vi "Impedance_Single_Meas.vi"(11 "Test Params Cluster":T1={"Test Freq. (Hz)"=1702.3933752476319, "Output Signal Amplitude\nVolts Pk"=0.1, "Sampling Time (s)"=0.01, "Sampling Rate (Hz)"=250000.0, "Output Channel"="Dev3/ao0", "Current Channel"="Dev3/ai1", "Voltage Channel"="Dev3/ai0", "Trigger Channel"="/Dev3/ao/StartTrigger", "Number of runs"=5}) -> (0 "Current Complex":cdb=0.1092230559688666-0.017870132117080606i, 1 "Voltage Complex":cdb=-0.17452167799153867-1.07754869267134i, 2 "Time domain Current":waveform(dbl)(graph)={"t0"=timestamp(3724535126.9386544 s since 1904-01-01), "dt"=3.999999999999989e-06, "Y"=array[2500 elements], "attributes"=variant("NI_ChannelName"=variant(string "Dev3/ai1"), "NI_UnitDescription"=variant(string "Volts"))}, 3 "Time domain Voltage":waveform(dbl)(graph)={"t0"=timestamp(3724535127.000671 s since 1904-01-01), "dt"=3.999999999999989e-06, "Y"=array[2500 elements], "attributes"=variant("NI_ChannelName"=variant(string "Dev3/ai0"), "NI_UnitDescription"=variant(string "Volts"))})   [LabVIEW 2020]
uses:
  <vilib>/measure/NI_MABase.lvlib
  <vilib>/DAQmx/configure/timing.llb/DAQmx Timing (Sample Clock).vi
  <vilib>/DAQmx/create/channels.llb/DAQmx Create Channel (AI-Voltage-Basic).vi
  <vilib>/DAQmx/read.llb/DAQmx Read (Analog 1D Wfm NChan NSamp).vi
  <vilib>/DAQmx/configure/trigger.llb/DAQmx Start Trigger (Digital Edge).vi
  <vilib>/DAQmx/create/channels.llb/DAQmx Create Channel (AO-Voltage-Basic).vi
  <vilib>/DAQmx/write.llb/DAQmx Write (Analog Wfm 1Chan NSamp).vi
  <vilib>/measure/NI_MAPro.lvlib
  <vilib>/measure/matone.llb/Extract Single Tone Information 1 Chan.vi
panel:
  out "Test Freq. (Hz)":dbl=1702.3933752476319
  out "Mag Current":dbl=0.1106752798824565
  in  "Use LabView\nSignal Detect":bool=TRUE
  out "detected phase (Rad)":dbl=4.551821517545998
  out "detected amplitude":dbl=1.0915901250774929 format="%.2p"
  in  "search (+/- % of Fsampl.)":dbl
  in  "advanced search":T2={"approx freq. (optional)"=-1.0, "search (+/- % of Fsampl.)"=5.0} {"search (+/- % of Fsampl.)" format="%0.2p"; "approx freq. (optional)" format="%0.2p"}
  out "Detected Time domain Current 2":waveform(dbl)(graph)={"t0"=timestamp(2.12 s since 1904-01-01), "dt"=4e-06, "Y"=array[2500 elements]}
  out "Detected Time domain Voltage 2":waveform(dbl)(graph)={"t0"=timestamp(2.13 s since 1904-01-01), "dt"=4e-06, "Y"=array[2500 elements]}
  out "detected frequency 2":dbl=1700.0000000000045 format="%.2p"
  out "detected frequency":dbl=1700.0000000000045 format="%.2p"
  out "Current phase (deg)":dbl=-0.16217447631966198 format="%.2p"
  out "Voltage phase (deg)":dbl=260.8001620522193 format="%.2p"
  in  "CurentRangeMax":dbl=5.0 format="%0.2f"
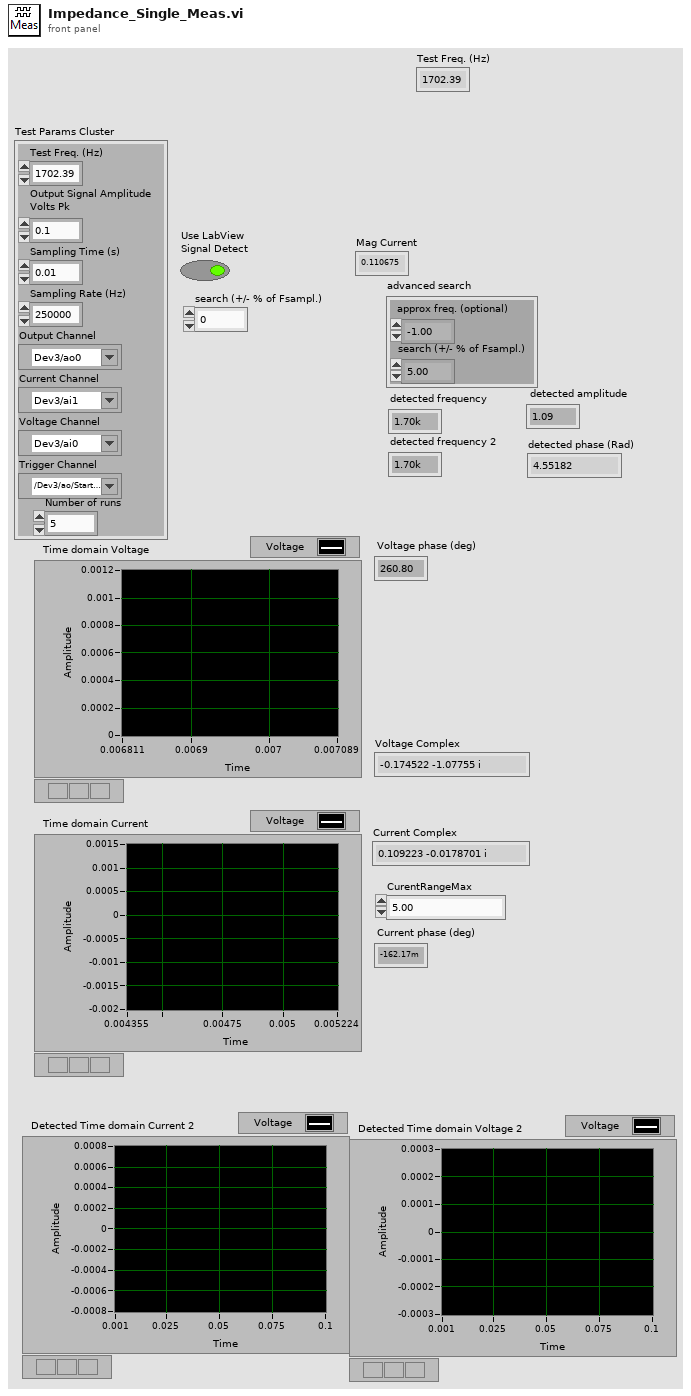
[diagram p1: front panel]
types:
  T1 = cluster{"Test Freq. (Hz)":dbl, "Output Signal Amplitude\nVolts Pk":dbl, "Sampling Time (s)":dbl, "Sampling Rate (Hz)":dbl, "Output Channel":tag, "Current Channel":tag, "Voltage Channel":tag, "Trigger Channel":tag, "Number of runs":i32}
  T2 = cluster{"approx freq. (optional)":dbl, "search (+/- % of Fsampl.)":dbl}
  T3 = enum32{"none", "input signal", "detected signal", "residual signal"}
  T4 = cluster{"exported time signal":waveform(dbl), "exported spectrum (dB)":cluster{"f0":dbl, "df":dbl, "dB Spectrum (Hann)":dbl[]}}
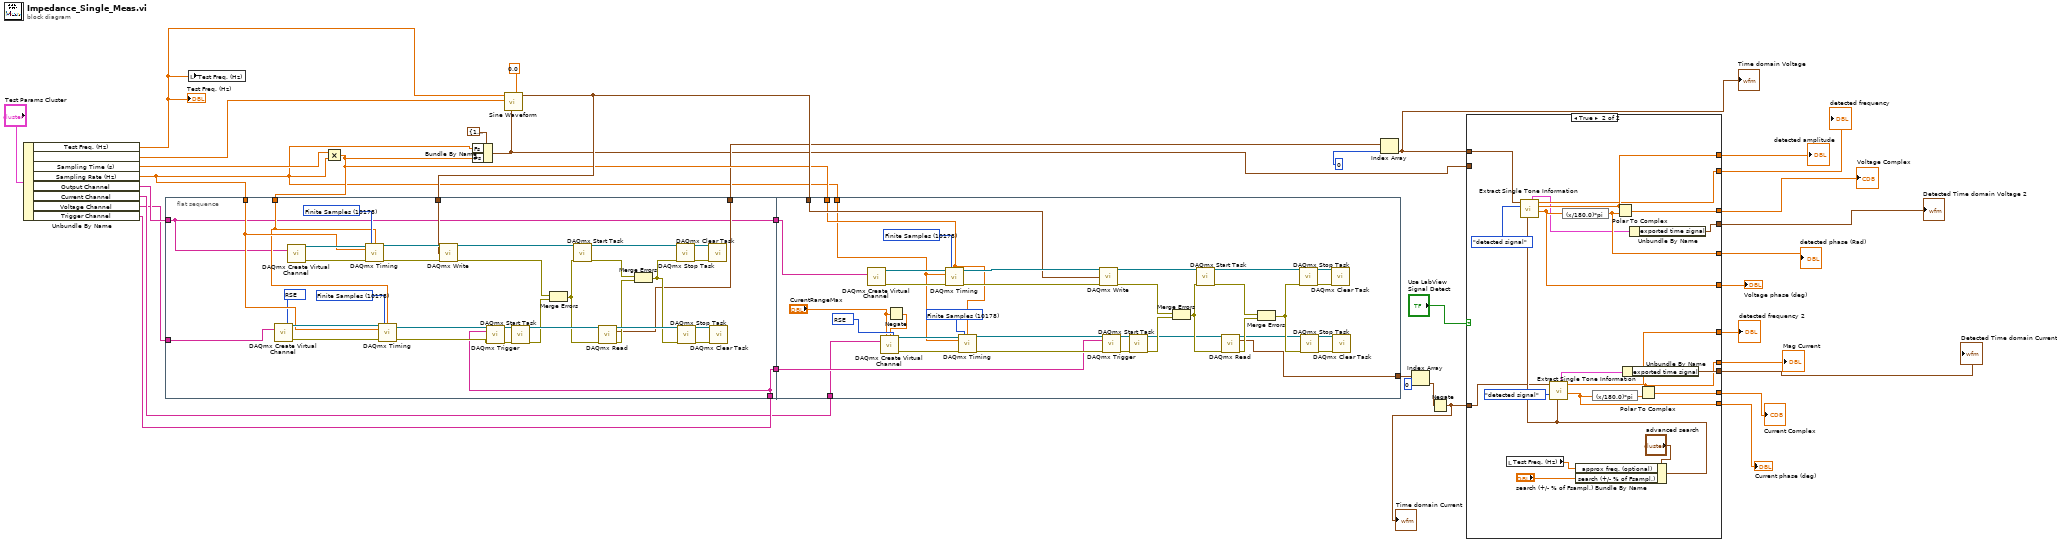
[diagram p0: block diagram]
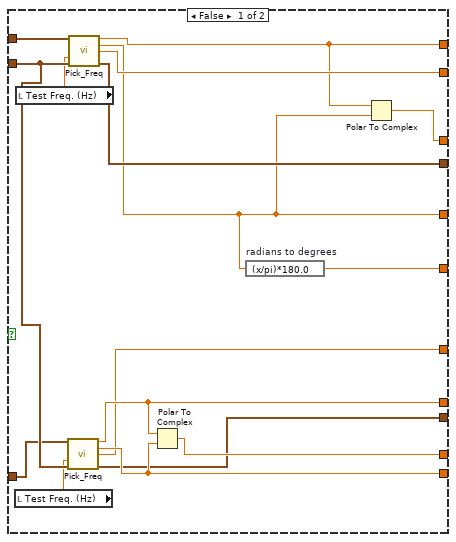
[diagram p2: hidden frame]
diagram:
  n1 = Unbundle By Name("Test Params Cluster") -> ("Test Freq. (Hz)"=w8:dbl, "Output Signal Amplitude\nVolts Pk"=w7:dbl, "Sampling Time (s)"=w6:dbl, "Sampling Rate (Hz)"=w5:dbl, "Output Channel"=w3:tag, "Current Channel"=w2:tag, "Voltage Channel"=w1:tag, "Trigger Channel"=w4:tag)
  "Test Freq. (Hz)" <- w8
  n2 = flat-sequence {
    tunnel: w5 -> [w47]
    tunnel: w31 -> [w46]
    tunnel: w32 -> [w44]
    tunnel: [w39] -> w28
    tunnel: [w38] -> w33
    tunnel: [w36] -> w21
    tunnel: w3 -> [w38]
    tunnel: w1 -> [w37]
    tunnel: w4 -> [w36]
    tunnel: w33 -> [w78]
    tunnel: [w77] -> w25
    tunnel: w32 -> [w76]
    tunnel: w31 -> [w75]
    tunnel: w5 -> [w74]
    tunnel: w21 -> [w71]
    tunnel: w2 -> [w70]
    frame #0 {
      w45 = 10083 items=["Default"=-1, "RSE"=10083, "NRSE"=10078, "Differential"=10106, "Pseudodifferential"=12529] ("input terminal configuration")
      w59 = 10178 items=["Finite Samples"=10178, "Continuous Samples"=10123, "Hardware Timed Single Point"=12522] ("sample mode")
      w62 = 10178 items=["Finite Samples"=10178, "Continuous Samples"=10123, "Hardware Timed Single Point"=12522] ("sample mode")
      n3 = call-poly <vilib>:"DAQmx Create Virtual Channel.vi"("input terminal configuration"=w45, "physical channels"=w37) -> ("task out"=w60:refnum<k21>, "error out"=w61:errorcluster)  [unwired: 12 in]
      n4 = call-poly <vilib>:"DAQmx Create Virtual Channel.vi"("physical channels"=w38) -> ("task out"=w69:refnum<k21>, "error out"=w65:errorcluster)  [unwired: 13 in]
      n5 = call-poly <vilib>:"DAQmx Timing.vi"("task/channels in"=w69, "sample mode"=w62, "samples per channel"=w46, "rate"=w47, "error in"=w65) -> ("task out"=w68:refnum<k21>, "error out"=w66:errorcluster)  [unwired: 9 in]
      n6 = call-poly <vilib>:"DAQmx Timing.vi"("task/channels in"=w60, "sample mode"=w59, "samples per channel"=w46, "rate"=w47, "error in"=w61) -> ("task out"=w58:refnum<k21>, "error out"=w57:errorcluster)  [unwired: 9 in]
      n7 = call-poly <vilib>:"DAQmx Write.vi"("task/channels in"=w68, "data"=w44, "error in"=w66) -> ("task out"=w67:refnum<k21>, "error out"=w49:errorcluster)  [unwired: 10 in, 1 out]
      n8 = call-poly <vilib>:"DAQmx Trigger.vi"("task/channels in"=w58, "source"=w36, "error in"=w57) -> ("task out"=w55:refnum<k21>, "error out"=w56:errorcluster)  [unwired: 11 in]
      n9 = call <vilib>:"DAQmx Start Task.vi"("task/channels in"=w55, "error in"=w56) -> ("task out"=w54:refnum<k21>, "error out"=w50:errorcluster)  [unwired: 12 in]
      n10 = Merge Errors(w49, w50) -> (w48:errorcluster)
      n11 = call <vilib>:"DAQmx Start Task.vi"("task/channels in"=w67, "error in"=w48) -> ("task out"=w64:refnum<k21>, "error out"=w41:errorcluster)  [unwired: 12 in]
      n12 = call-poly <vilib>:"DAQmx Read.vi"("task/channels in"=w54, "error in"=w48) -> ("task out"=w51:refnum<k21>, "data"=w39:waveform(dbl)[], "error out"=w42:errorcluster)  [unwired: 11 in]
      n13 = Merge Errors(w41, w42) -> (w40:errorcluster)
      n14 = call <vilib>:"DAQmx Stop Task.vi"("task/channels in"=w64, "error in"=w40) -> ("task out"=w63:refnum<k21>, "error out"=w43:errorcluster)  [unwired: 12 in]
      n15 = call <vilib>:"DAQmx Stop Task.vi"("task/channels in"=w51, "error in"=w40) -> ("task out"=w52:refnum<k21>, "error out"=w53:errorcluster)  [unwired: 12 in]
      n16 = call <vilib>:"DAQmx Clear Task.vi"("task in"=w63, "error in"=w43) -> ()  [unwired: 13 in, 1 out]
      n17 = call <vilib>:"DAQmx Clear Task.vi"("task in"=w52, "error in"=w53) -> ()  [unwired: 13 in, 1 out]
    }
    frame #1 {
      w101 = 10083 items=["Default"=-1, "RSE"=10083, "NRSE"=10078, "Differential"=10106, "Pseudodifferential"=12529] ("input terminal configuration")
      w89 = 10178 items=["Finite Samples"=10178, "Continuous Samples"=10123, "Hardware Timed Single Point"=12522] ("sample mode")
      w86 = 10178 items=["Finite Samples"=10178, "Continuous Samples"=10123, "Hardware Timed Single Point"=12522] ("sample mode")
      n18 = call-poly <vilib>:"DAQmx Create Virtual Channel.vi"("physical channels"=w78) -> ("task out"=w79:refnum<k21>, "error out"=w83:errorcluster)  [unwired: 13 in]
      n19 = Negate(x="CurentRangeMax") -> (-x=w72:dbl)
      n20 = call-poly <vilib>:"DAQmx Create Virtual Channel.vi"("maximum value"="CurentRangeMax", "minimum value"=w72, "input terminal configuration"=w101, "physical channels"=w70) -> ("task out"=w88:refnum<k21>, "error out"=w87:errorcluster)  [unwired: 10 in]
      n21 = call-poly <vilib>:"DAQmx Timing.vi"("task/channels in"=w79, "sample mode"=w86, "samples per channel"=w75, "rate"=w74, "error in"=w83) -> ("task out"=w80:refnum<k21>, "error out"=w82:errorcluster)  [unwired: 9 in]
      n22 = call-poly <vilib>:"DAQmx Timing.vi"("task/channels in"=w88, "sample mode"=w89, "samples per channel"=w75, "rate"=w74, "error in"=w87) -> ("task out"=w90:refnum<k21>, "error out"=w91:errorcluster)  [unwired: 9 in]
      n23 = call-poly <vilib>:"DAQmx Write.vi"("task/channels in"=w80, "data"=w76, "error in"=w82) -> ("task out"=w81:refnum<k21>, "error out"=w99:errorcluster)  [unwired: 10 in, 1 out]
      n24 = call-poly <vilib>:"DAQmx Trigger.vi"("task/channels in"=w90, "source"=w71, "error in"=w91) -> ("task out"=w93:refnum<k21>, "error out"=w92:errorcluster)  [unwired: 11 in]
      n25 = call <vilib>:"DAQmx Start Task.vi"("task/channels in"=w93, "error in"=w92) -> ("task out"=w94:refnum<k21>, "error out"=w98:errorcluster)  [unwired: 12 in]
      n26 = Merge Errors(w99, w98) -> (w100:errorcluster)
      n27 = call <vilib>:"DAQmx Start Task.vi"("task/channels in"=w81, "error in"=w100) -> ("task out"=w84:refnum<k21>, "error out"=w104:errorcluster)  [unwired: 12 in]
      n28 = call-poly <vilib>:"DAQmx Read.vi"("task/channels in"=w94, "error in"=w100) -> ("task out"=w97:refnum<k21>, "data"=w77:waveform(dbl)[], "error out"=w103:errorcluster)  [unwired: 11 in]
      n29 = Merge Errors(w104, w103) -> (w105:errorcluster)
      n30 = call <vilib>:"DAQmx Stop Task.vi"("task/channels in"=w84, "error in"=w105) -> ("task out"=w85:refnum<k21>, "error out"=w102:errorcluster)  [unwired: 12 in]
      n31 = call <vilib>:"DAQmx Stop Task.vi"("task/channels in"=w97, "error in"=w105) -> ("task out"=w96:refnum<k21>, "error out"=w95:errorcluster)  [unwired: 12 in]
      n32 = call <vilib>:"DAQmx Clear Task.vi"("task in"=w85, "error in"=w102) -> ()  [unwired: 13 in, 1 out]
      n33 = call <vilib>:"DAQmx Clear Task.vi"("task in"=w96, "error in"=w95) -> ()  [unwired: 13 in, 1 out]
    }
  }
  n34 = local write "Test Freq. (Hz)"(w8) -> ()
  n35 = Multiply(x=w6, y=w5) -> (x*y=w31:dbl)
  n36 = Bundle By Name(cluster=cluster{"Fs":dbl, "#s":dbl} {"Fs"=1000.0, "#s"=1000.0} ("sampling info"), "Fs"=w5, "#s"=w31) -> (w11:cluster{"Fs":dbl, "#s":dbl})
  n37 = call <vilib>:"Sine Waveform.vi"("offset"=0.0, "sampling info"=w11, "amplitude"=w7, "frequency"=w8) -> ("signal out"=w32:waveform(dbl))  [unwired: 6 in, 1 out]
  n38 = Index Array(array=w28, index=0) -> (element=w20:waveform(dbl))
  "Time domain Voltage" <- w20
  n39 = Index Array(array=w25, index=0) -> (element=w23:waveform(dbl))
  n40 = Negate(x=w23) -> (-x=w10:waveform(dbl))
  "Time domain Current" <- w10
  n41 = case shown="True" "Use LabView\nSignal Detect" {
    tunnel: [w111 w143] -> w30
    tunnel: [w110 w142] -> w29
    tunnel: [w112 w140] -> w24
    tunnel: [w120 w139] -> w22
    tunnel: w20 -> [w121 w133]
    tunnel: [w114 w132] -> w18
    tunnel: [w117 w131] -> w17
    tunnel: [w118 w130] -> w16
    tunnel: [w113 w129] -> w15
    tunnel: [w119 w124] -> w14
    tunnel: [w115 w126] -> w13
    tunnel: [w116 w125] -> w12
    tunnel: w11 -> [w109 _]
    tunnel: w10 -> [w108 w123]
    frame False {
      n42 = local read "Test Freq. (Hz)"() -> (w107:dbl)
      n43 = local read "Test Freq. (Hz)"() -> (w106:dbl)
      n44 = call "Pick_Freq.vi"("time signal"=w108, "RX frequency"=w107, "sampling info"=w109) -> ("Mag"=w119:dbl, "Phase"=w118:dbl, "actual freq"=w114:dbl, "signal out"=w115:waveform(dbl))  [unwired: 9 in]
      n45 = call "Pick_Freq.vi"("time signal"=w121, "RX frequency"=w106, "sampling info"=w109) -> ("Mag"=w111:dbl, "Phase"=w110:dbl, "actual freq"=w120:dbl, "signal out"=w116:waveform(dbl))  [unwired: 9 in]
      n46 = Polar To Complex(1:w118, 2:w119) -> (0:w117:cdb)
      n47 = expression code="(x/pi)*180.0" "radians to degrees"(w110) -> (w113:dbl)
      n48 = Polar To Complex(1:w110, 2:w111) -> (0:w112:cdb)
    }
    frame True {
      n49 = local read "Test Freq. (Hz)"() -> (w122:dbl)
      n50 = Bundle By Name(cluster="advanced search", "approx freq. (optional)"=w122, "search (+/- % of Fsampl.)"="search (+/- % of Fsampl.)") -> (w135:T2)
      n51 = call-poly <vilib>:"Extract Single Tone Information.vi"("advanced search"=w135, "export mode"=T3."detected signal", "time signal in"=w133) -> ("detected phase (deg)"=w129:dbl, "detected amplitude"=w143:dbl, "detected frequency"=w139:dbl, "exported signals"=w128:T4)  [unwired: 3 in, 2 out]
      n52 = call-poly <vilib>:"Extract Single Tone Information.vi"("advanced search"=w135, "export mode"=T3."detected signal", "time signal in"=w123) -> ("detected phase (deg)"=w130:dbl, "detected amplitude"=w124:dbl, "detected frequency"=w132:dbl, "exported signals"=w127:T4)  [unwired: 3 in, 2 out]
      n53 = expression code="(x/180.0)*pi" ("degrees to radians")(w129) -> (w142:dbl)
      n54 = expression code="(x/180.0)*pi" ("degrees to radians")(w130) -> (w141:dbl)
      n55 = Polar To Complex(1:w142, 2:w143) -> (0:w140:cdb)
      n56 = Unbundle By Name(w127) -> ("exported time signal"=w126:waveform(dbl))
      n57 = Unbundle By Name(w128) -> ("exported time signal"=w125:waveform(dbl))
      n58 = Polar To Complex(1:w141, 2:w124) -> (0:w131:cdb)
    }
  }
  "Voltage Complex" <- w24
  "detected frequency" <- w22
  "Detected Time domain Voltage 2" <- w12
  "Detected Time domain Current 2" <- w13
  "detected amplitude" <- w30
  "detected phase (Rad)" <- w29
  "detected frequency 2" <- w18
  "Current Complex" <- w17
  "Current phase (deg)" <- w16
  "Voltage phase (deg)" <- w15
  "Mag Current" <- w14
